vi "Safety Box.vi"(4 "Right\n in":bool, 5 "Left Limit In":bool, 6 "Left in":bool, 7 "Right Limit":bool, 8 "Up in":bool, 9 "Down in":bool, 10 "Up Limit":bool, 11 "Down limit":bool) -> (0 "Left out":bool, 1 "Right out":bool, 2 "Up Out":bool, 3 "Down out":bool)   [LabVIEW 2015]
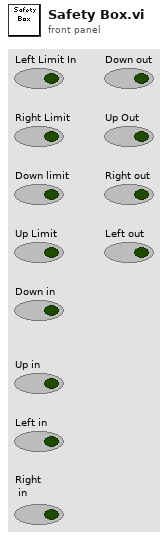
[diagram p1: front panel]
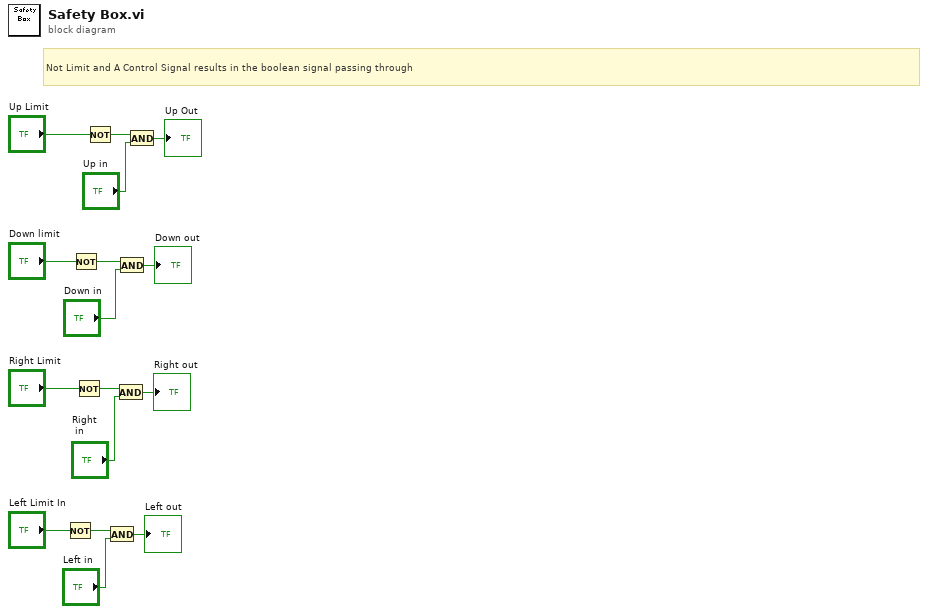
[diagram p0: block diagram]
diagram:
  # "Not Limit and A Control Signal results in the boolean signal passing through"
  n1 = Not(x="Left Limit In") -> (.not. x?=w5:bool)
  n2 = Not(x="Down limit") -> (.not. x?=w1:bool)
  n3 = Not(x="Right Limit") -> (.not. x?=w7:bool)
  n4 = Not(x="Up Limit") -> (.not. x?=w3:bool)
  n5 = And(x=w5, y="Left in") -> (x .and. y?=→"Left out":bool)
  n6 = And(x=w7, y="Right\n in") -> (x .and. y?=→"Right out":bool)
  n7 = And(x=w1, y="Down in") -> (x .and. y?=→"Down out":bool)
  n8 = And(x=w3, y="Up in") -> (x .and. y?=→"Up Out":bool)
